vi "Temperature Logger.vi"() -> ()   [LabVIEW 2012]
uses:
  <vilib>/Analysis/NI_AALBase.lvlib
  <vilib>/Analysis/baseanly.llb/Mean (DBL).vi
panel:
  out "Max":i32
  out "Min":dbl
  out "Mean":i32
  in  "stop 2":bool
  out "Current Data Point":dbl
  out "?":dbl
  in  "Current Data":dbl(slide) scale=0.0..10.0
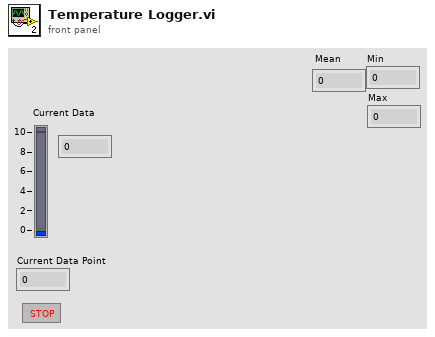
[diagram p1: front panel]
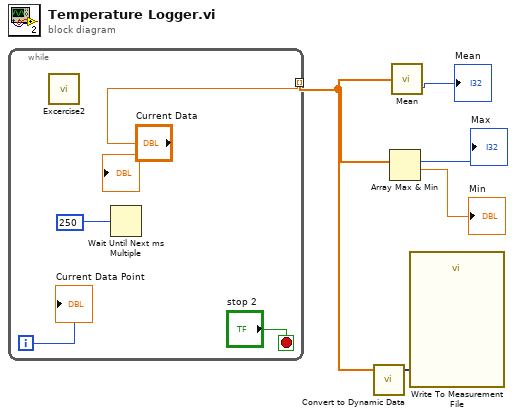
[diagram p0: block diagram]
diagram:
  n1 = while {
    tunnel: ["Current Data"] -> w2 mode=indexing
    i -> [w8]
    stop <- "stop 2" stop-if-true
    n2 = call "Excercise2.vi"() -> ()  [unwired: 12 in]
    n3 = Wait Until Next ms Multiple(millisecond multiple=250) -> ()  [unwired: 1 out]
    "Current Data Point" <- w8
  }
  n4 = call "Convert to Dynamic Data"("Array"=w2) -> ("Dynamic Data Type"=w1:dynamicdata)  [unwired: 3 in]
  n5 = Array Max & Min(array=w2) -> (max index (indices)=→"Max":i32, min value=→"Min":dbl)  [unwired: 2 out]
  n6 = call-poly <vilib>:"Mean.vi"("X"=w2) -> ("error"=→"Mean":i32)  [unwired: 1 out]
  n7 = call "Write To Measurement File"("Signals"=w1) -> ()  [unwired: 16 in, 3 out]
